vi "Get_Input.vi"(8 "error in (no error)":errorcluster, 11 "FrontPanelData in":refnum<class "EpiWrapper.lvclass">) -> (0 "error out":errorcluster, 2 "Input":refnum<vi>, 3 "FrontPanelData out":refnum<class "EpiWrapper.lvclass">)   [LabVIEW 2012, in "EpiWrapper.lvclass"]
uses:
  EpiWrapper.lvclass
  EpiWrapper.lvclass/EpiWrapper.ctl
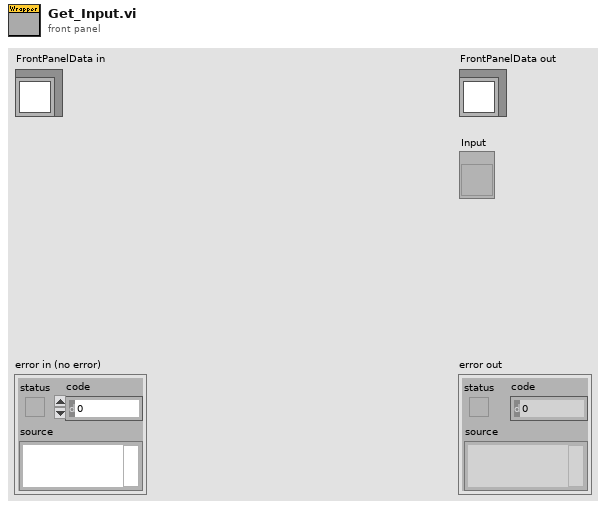
[diagram p1: front panel]
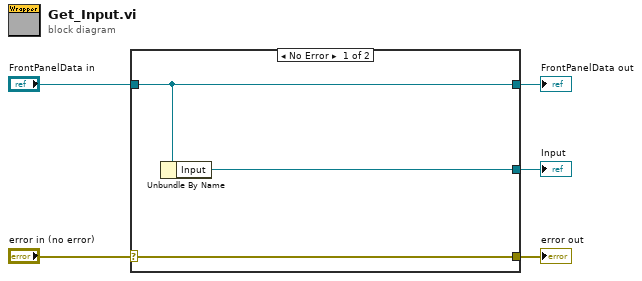
[diagram p0: block diagram]
diagram:
  n1 = case shown="No Error" "error in (no error)" {
    selector: "error in (no error)" -> [w8 w9]
    tunnel: [w8 w9] -> w4
    tunnel: [w7 w10] -> w2
    tunnel: "FrontPanelData in" -> [w7 w10]
    tunnel: [w6 _] -> w1
    frame No Error {
      n2 = Unbundle By Name(w7) -> ("Input"=w6:refnum<vi>)
    }
    frame Error {
    }
  }
  "error out" <- w4
  "FrontPanelData out" <- w2
  "Input" <- w1
